vi "Load dynam called VIs.vi"   [LabVIEW 2013]
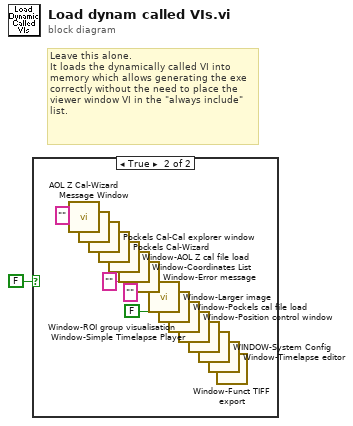
[diagram p0: block diagram]
diagram:
  # "Leave this alone.\nIt loads the dynamically called VI into memory which allows generating the exe correctly without the need to place the viewer window VI in the \"always include\" list."
  n1 = case shown="True" FALSE {
    frame False {
    }
    frame True {
      n2 = call "AOL Z Cal-Wizard.vi"() -> ()  [unwired: 12 in]
      n3 = call "Message Window.vi"("Message string"="") -> ()  [unwired: 10 in, 1 out]
      n4 = call "Pockels Cal-Cal explorer window.vi"() -> ()  [unwired: 12 in]
      n5 = call "Pockels Cal-Wizard.vi"() -> ()  [unwired: 12 in]
      n6 = call "Window-AOL Z cal file load.vi"() -> ()  [unwired: 12 in]
      n7 = call "Window-Coordinates List.vi"() -> ()  [unwired: 12 in]
      n8 = call "Window-Error message.vi"("Message"="") -> ()  [unwired: 10 in, 1 out]
      n9 = call "Window-Larger image.vi"("Image name"="", "Open maximised"=FALSE) -> ()  [unwired: 10 in]
      n10 = call "Window-Pockels cal file load.vi"() -> ()  [unwired: 12 in]
      n11 = call "Window-Position control window.vi"() -> ()  [unwired: 12 in]
      n12 = call "Window-ROI group visualisation.vi"() -> ()  [unwired: 11 in, 1 out]
      n13 = call "Window-Simple Timelapse Player.vi"() -> ()  [unwired: 12 in]
      n14 = call "WINDOW-System Config.vi"() -> ()  [unwired: 12 in]
      n15 = call "Window-Timelapse editor.vi"() -> ()  [unwired: 12 in]
      n16 = call "Window-Funct TIFF export.vi"() -> ()  [unwired: 12 in]
    }
  }
